vi "TekAFG3102.vi"() -> ()   [LabVIEW 2015]
uses:
  NetworkStream/NetworkStreamReceiverState.ctl
  Shared program Control/loop state machine.ctl
  NetworkStream/NetworkStreamStateMachineVariable.ctl
  NetworkStream/NetworkStreamData.ctl
  Shared program Control/MasterStatus.ctl
  <vilib>/dex/Stream Element Allocation Mode.ctl
  ICcamera/MyToolsFunction.lvlib
  Tek shared libraries/ArbitraryFunctions.lvlib
  NetworkStream/NetworkStream.lvlib
  Shared program Control/MySharedVariables.lvlib
panel:
  out "sequence number":u64
  out "loop state machine":T1=enum."load user waveform"
  in  "Stop Button":bool
  in  "slot to load (update first)":i32(ring) items=["Slot 1", "Slot 2", "Slot 3", "Slot 4"]
  in  "channels":enum32{"active channel", ""}(radio)
  in  "Channel ON/OFF":bool
  out "Network Stream State Indicator":T2
  out "Session Hash":u64
  out "ready":bool=TRUE
  in  "force trigger":bool
  in  "user waveform":bool
  in  "Tab Control":enum32{"CW", "AM", "FM", "PM", "Sweep", "Burst"}(tab)
  in  "CM cluster":T3={"Frequency (Hz)"=80000000.0, "Amplitude (V)"=0.2, "Phase (°)"=0.0, "Offset (Volt)"=0.0, "Standard waveform (1: Sine)"=1, "output mode"=0, "Modulation Waveform (1: Sine)"=1} {"Modulation Waveform (1: Sine)" items=["Sine"=1, "Square"=2, "Triangle"=3, "Ramp Up"=4, "Ramp Down"=5, "Noise"=100, "Arbitrary User1"=200, "Arbitrary User2"=201, "Arbitrary User3"=202, "Arbitrary User4"=203, "Edit Memory"=204]; "output mode" items=["Standard Function", "Arbitrary Waveform"]; "Standard waveform (1: Sine)" items=["Sine"=1, "Square"=2, "Pulse"=1002, "Ramp"=1001, "Noise"=1003, "DC"=6, "Sin(x)/x"=1004, "Gaussian"=1005, "Lorentz"=1006, "Exponential Rise"=1007, "Exponential Decay"=1008, "Haversine"=1009]}
  in  "AM Modulation Mode Cluster":T4={"waveform (1: Sine)"=1, "depth M (%)"=50.0, "Modulation source"=0, "AM Frequency (Hz)"=10.0, "ON/OFF"=FALSE} {"Modulation source" items=["Intern", "Extern"]; "waveform (1: Sine)" items=["Sine"=1, "Square"=2, "Pulse"=1002, "Ramp"=1001, "Noise"=1003, "DC"=6, "Sin(x)/x"=1004, "Gaussian"=1005, "Lorentz"=1006, "Exponential Rise"=1007, "Exponential Decay"=1008, "Haversine"=1009]}
  in  "FM":T5={"ON/OFF"=FALSE, "source (0: Internal)"=0, "peak deviation (1000000)"=1000000.0, "modulation frequency (10000)"=10000.0, "waveform (1: Sine)"=1} {"waveform (1: Sine)" items=["Sine"=1, "Square"=2, "Pulse"=1002, "Ramp"=1001, "Noise"=1003, "DC"=6, "Sin(x)/x"=1004, "Gaussian"=1005, "Lorentz"=1006, "Exponential Rise"=1007, "Exponential Decay"=1008, "Haversine"=1009]; "source (0: Internal)" items=["Internal", "External"]}
  in  "PM Modulation Cluster":T6={"Source (0: Internal)"=0, "Peak Deviation (90)"=90.0, "ON/OFF"=FALSE, "Modulation Frequency (10000)"=10000.0, "Modulation Waveform (1: Sine)"=1} {"Modulation Waveform (1: Sine)" items=["Sine"=1, "Square"=2, "Triangle"=3, "Ramp Up"=4, "Ramp Down"=5, "Noise"=100, "Arbitrary User1"=200, "Arbitrary User2"=201, "Arbitrary User3"=202, "Arbitrary User4"=203, "Edit Memory"=204]; "Source (0: Internal)" items=["Internal", "External"]}
  in  "resource name":refnum<k15>
  # "By default, Define User Waveform will assume \na modulation frequency = PM. However, the \nvalue has no effect on sent data to controlor and \nis purely arbitrary"
  # "Depth M is varied between 0% and 120% (the latter corresponding \nto a maximum amplitude of A(Vpp)). Cf p63 doc"
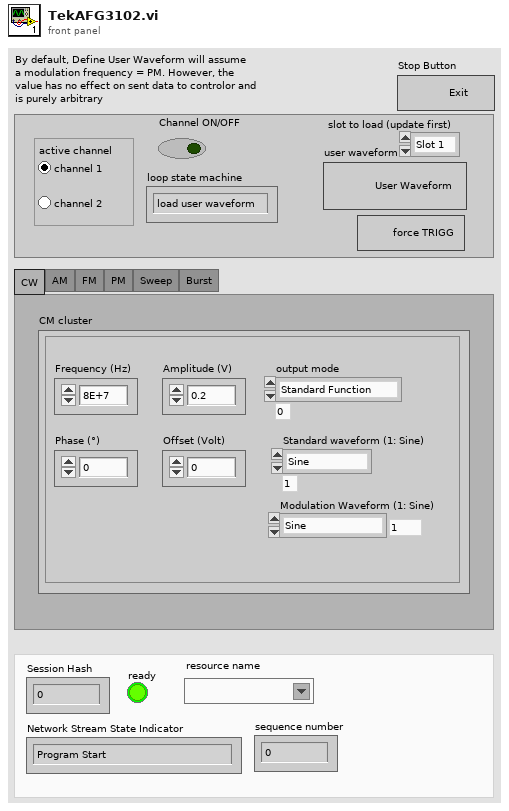
[diagram p1: front panel]
types:
  T1 = typedef "loop state machine.ctl" = enum16{"ready", "write on VISA", "get tek param", "load user waveform", "update channel parameters", "update status", "channel on/off", "initialize", "exit", "error"}
  T2 = typedef "NetworkStream.lvlib/NetworkStreamReceiverState.ctl" = enum16{"Program Start", "Waiting for connection", "Connected", "Connection lost", "Exit", "Unhandled Exception"}
  T3 = cluster{"Frequency (Hz)":dbl, "Amplitude (V)":dbl, "Phase (°)":dbl, "Offset (Volt)":dbl, "Standard waveform (1: Sine)":i32, "output mode":i32, "Modulation Waveform (1: Sine)":i32}
  T4 = cluster{"waveform (1: Sine)":i32, "depth M (%)":dbl, "Modulation source":u16, "AM Frequency (Hz)":dbl, "ON/OFF":bool}
  T5 = cluster{"ON/OFF":bool, "source (0: Internal)":i32, "peak deviation (1000000)":dbl, "modulation frequency (10000)":dbl, "waveform (1: Sine)":i32}
  T6 = cluster{"Source (0: Internal)":i32, "Peak Deviation (90)":dbl, "ON/OFF":bool, "Modulation Frequency (10000)":dbl, "Modulation Waveform (1: Sine)":i32}
  T7 = typedef "MySharedVariables.lvlib/MasterStatus.ctl" = cluster{"Camera done":bool, "Tektronik done":bool, "Motors done":bool, "Gage done":bool}[]
  T8 = typedef "NetworkStream.lvlib/NetworkStreamData.ctl" = cluster{"Command/Status":string, "Data":variant, "Session Hash":u64, "Sequence Number":u64}
  T9 = typedef "NetworkStream.lvlib/NetworkStreamStateMachineVariable.ctl" = cluster{"Network Stream Reader Endpoint":refnum<k21>, "Last Received Sequence Number":u64}
  T10 = cluster{"Frequency (Hz)":dbl, "Amplitude (V)":dbl, "Phase (°)":dbl, "Offset (Volt)":dbl, "waveform (1: Sine)":i32, "output mode":i32}
  T11 = cluster{"max number of waveforms":i32, "waveform quantum":i32, "max waveform size":i32, "min waveform size":i32}
  T12 = cluster{"Camera done":bool, "Tektronik done":bool, "Motors done":bool, "Gage done":bool}
  T13 = typedef "Stream Element Allocation Mode.ctl" = u32
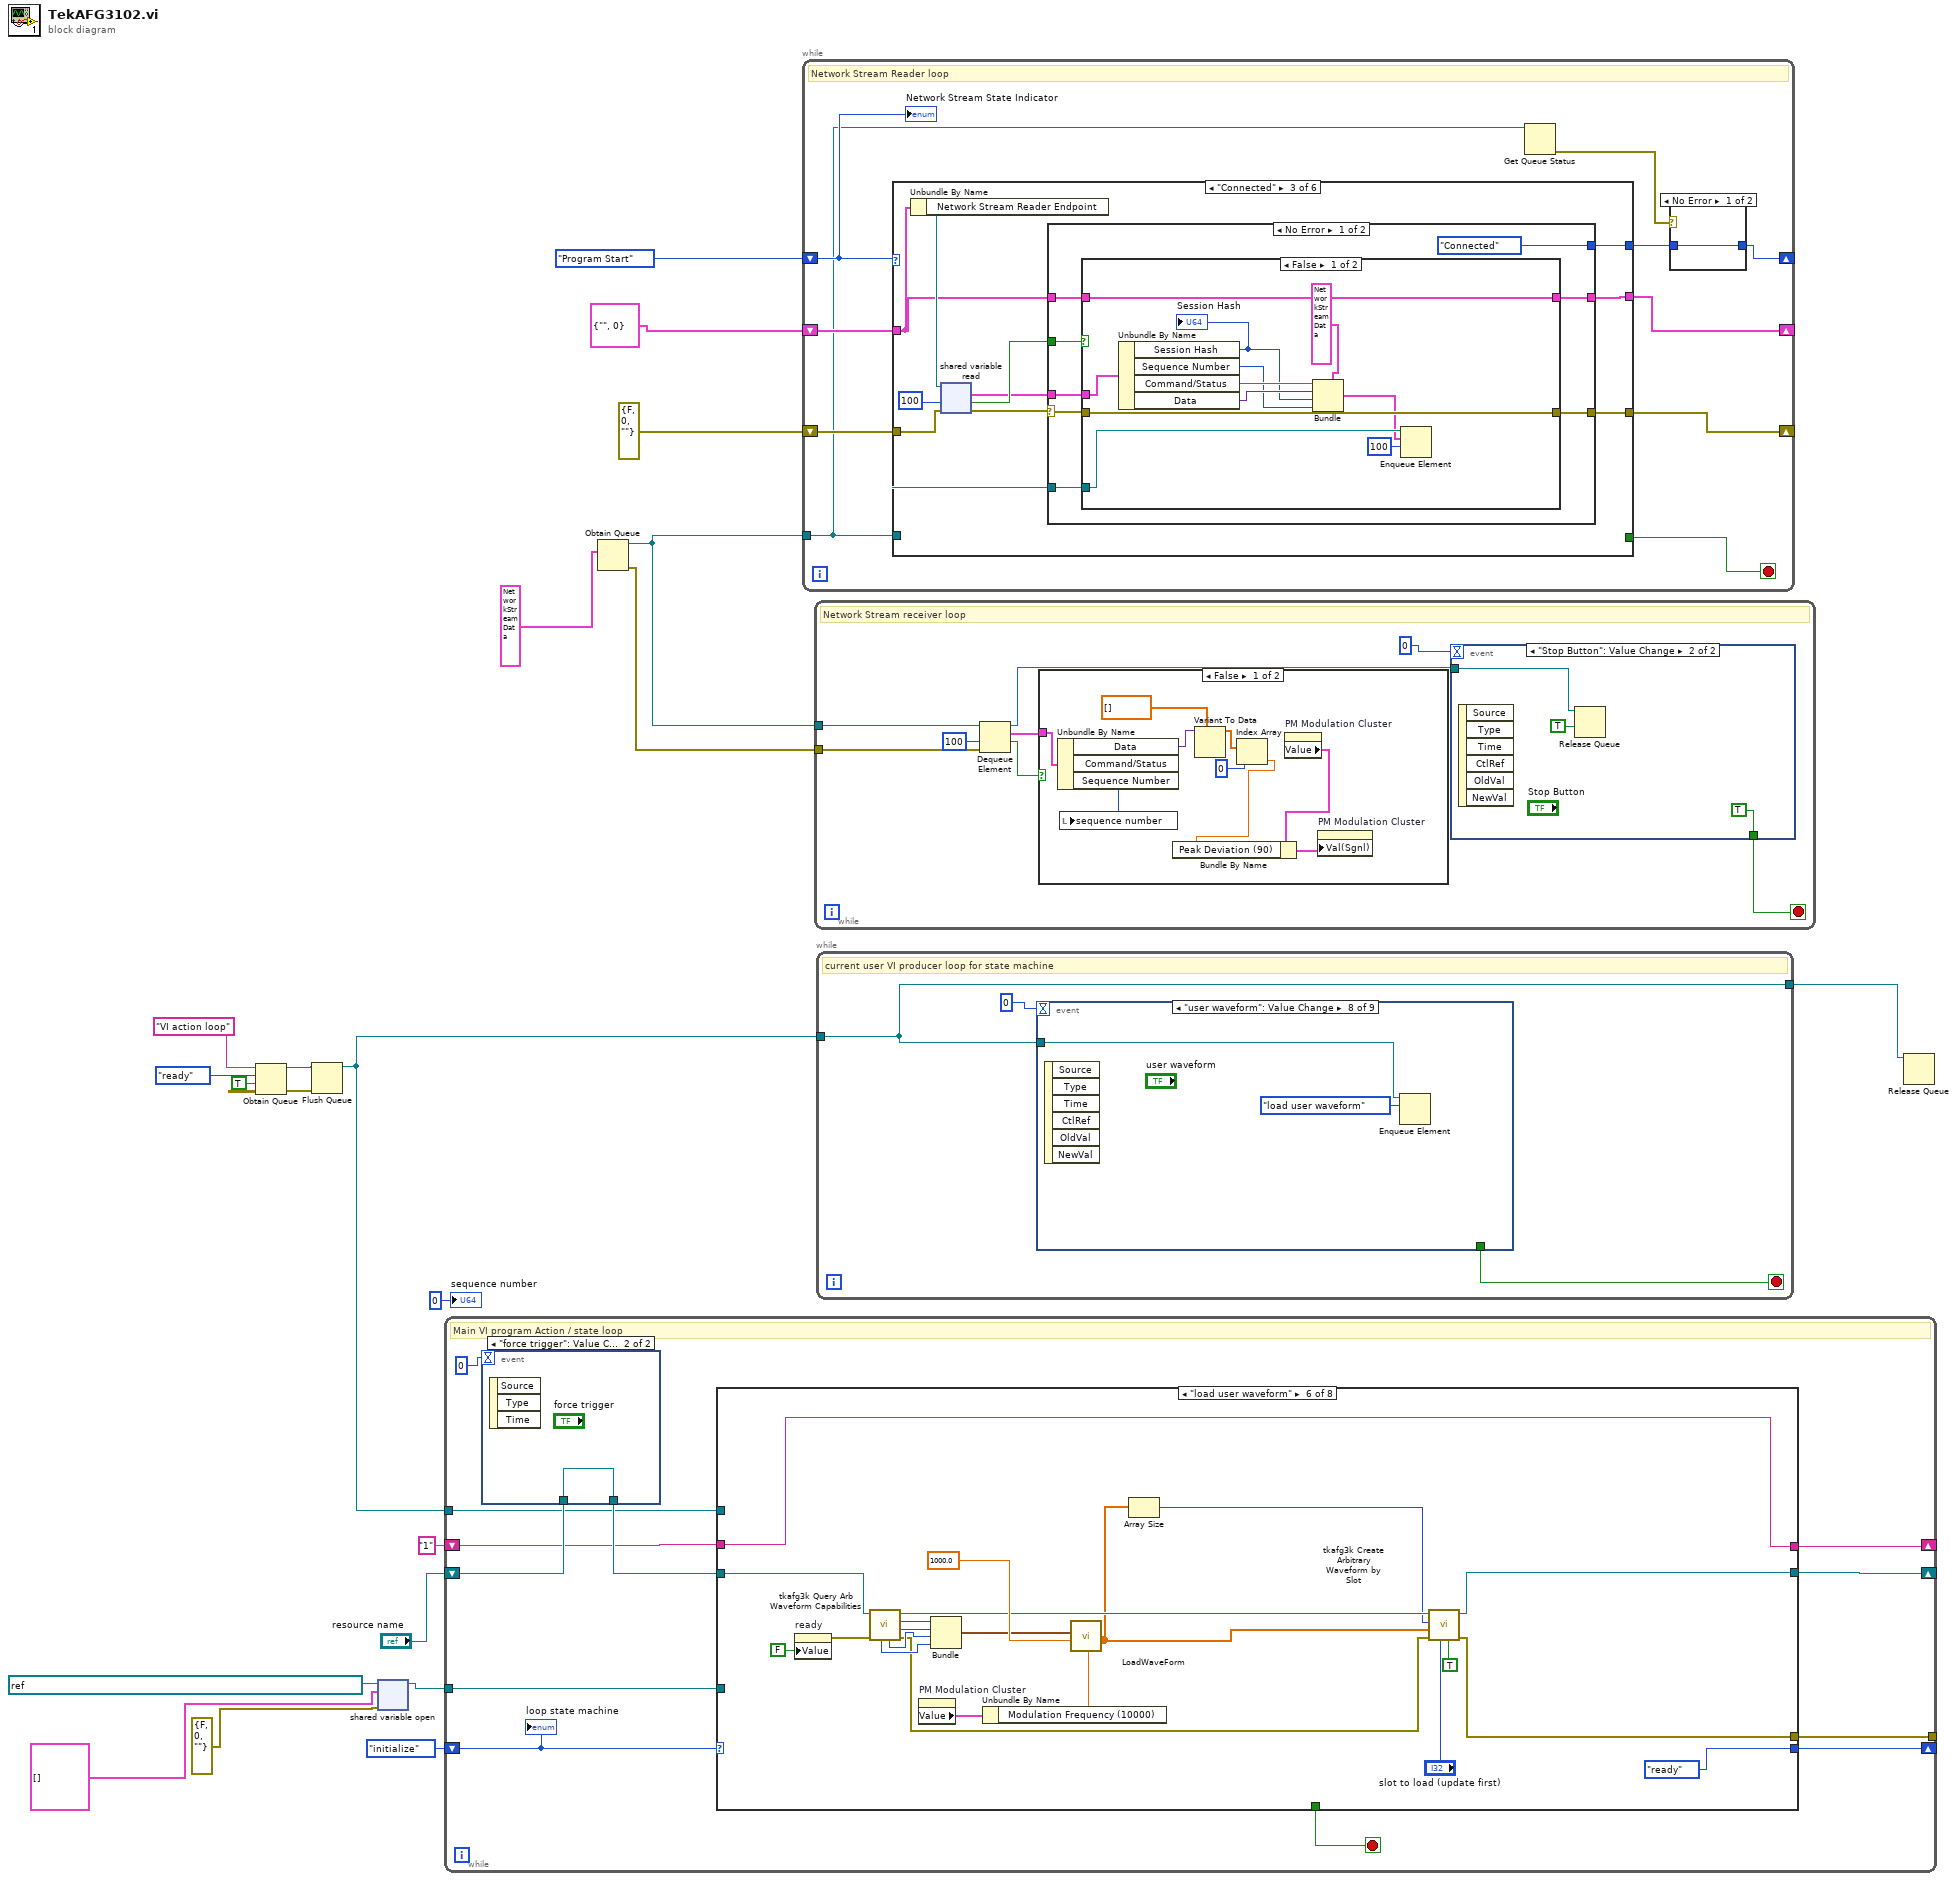
[diagram p0: block diagram]
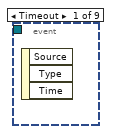
[diagram p2: hidden frame]
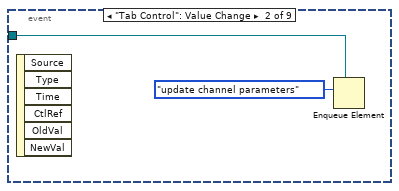
[diagram p3: hidden frame]
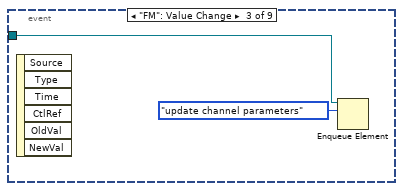
[diagram p4: hidden frame]
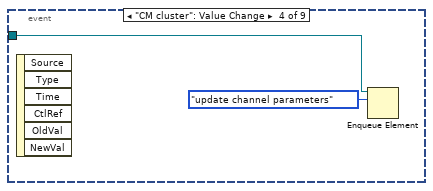
[diagram p5: hidden frame]
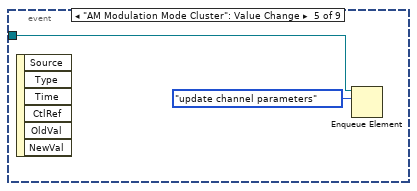
[diagram p6: hidden frame]
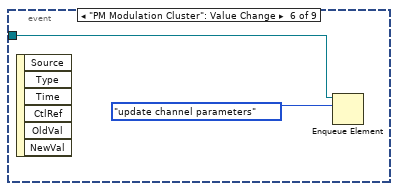
[diagram p7: hidden frame]
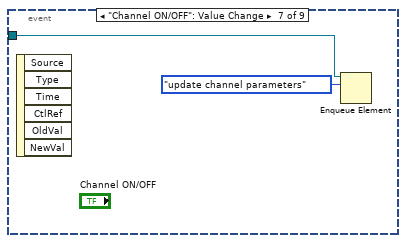
[diagram p8: hidden frame]
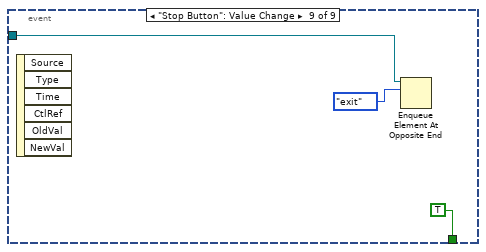
[diagram p9: hidden frame]
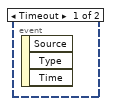
[diagram p11: hidden frame]
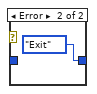
[diagram p12: hidden frame]
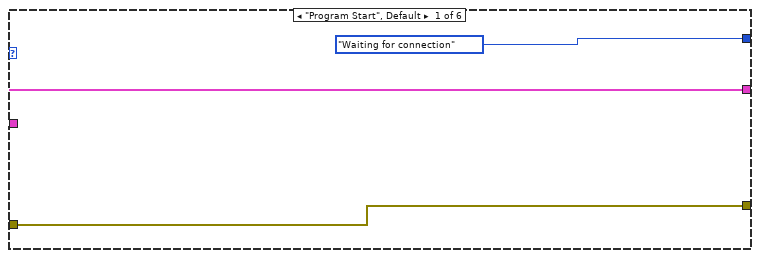
[diagram p13: hidden frame]
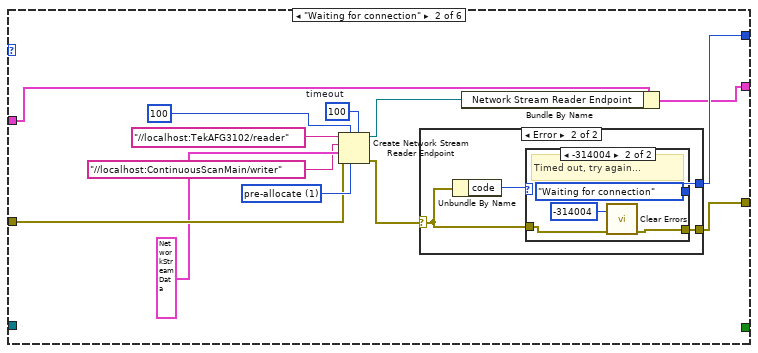
[diagram p14: hidden frame]
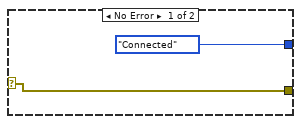
[diagram p15: hidden frame]
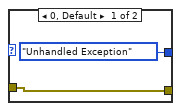
[diagram p16: hidden frame]
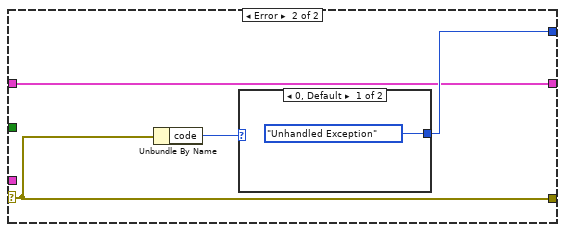
[diagram p18: hidden frame]
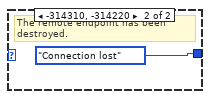
[diagram p19: hidden frame]
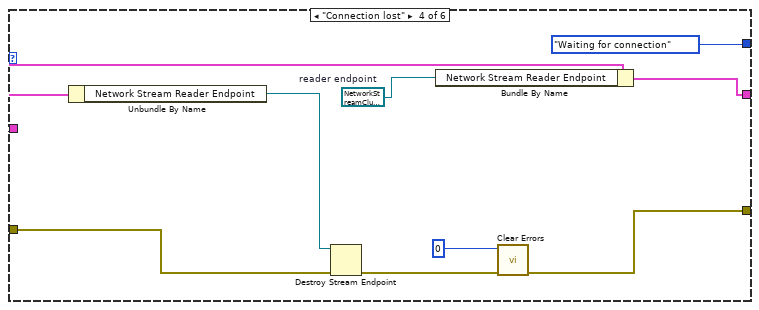
[diagram p20: hidden frame]
diagram:
  n1 = Obtain Queue(name (unnamed)="VI action loop", element data type=loop_state_machine."ready" ("loop state machine"), create if not found? (T)=TRUE) -> (queue out=w8:refnum<queue>, error out=w6:errorcluster)  [unwired: 2 in, 1 out]
  n2 = Flush Queue(queue=w8, error in (no error)=w6) -> (queue out=w7:refnum<queue>)  [unwired: 2 out]
  n3 = shared-variable-open(refnum<k21> "ni.var.psp://localhost/MySharedVariables/MasterStatusShared" ("shared variable refnum in"), errorcluster {"status"=FALSE, "code"=0, "source"=""} ("error in (no error)"), T7 [] ("MasterStatusShared")) -> (w3:refnum<k21>)  [unwired: 1 in, 1 out]
  n4 = while {
    tunnel: [w32] -> _
    shift-right: [w31] -> _
    shift-left: "resource name" -> [w26]
    shift-right: [w29] -> _
    shift-left: loop_state_machine."initialize" ("loop state machine") -> [w30]
    shift-right: [w27] -> _
    shift-left: "1" -> [w24]
    tunnel: w7 -> [w23]
    tunnel: w3 -> [w22]
    stop <- w33 stop-if-true
    # "Main VI program Action / state loop"
    n5 = event shown="[1] \"force trigger\": Value Change" {
      selector: _ -> [_ _]
      dyn-events: _ -> [_ _]
      timeout: 0 -> [_ _]
      tunnel: w26 -> [w34 w36]
      tunnel: [w34 w36] -> w25
      event Timeout {
        n6 = event-data() -> ()  [unwired: 1 in, 3 out]
        "ready" <- TRUE
      }
      event "force trigger": Value Change {
        n7 = event-data() -> ()  [unwired: 1 in, 3 out]
      }
    }
    n8 = case shown="\"load user waveform\"" w30 {
      tunnel: [_ TRUE _ _ _ _ _ _] -> w33
      tunnel: [w41 w54 errorcluster {"status"=FALSE, "code"=0, "source"=""} ("error out") errorcluster {"status"=FALSE, "code"=0, "source"=""} ("error out") w74 w134 w150 errorcluster {"status"=FALSE, "code"=0, "source"=""} ("error out")] -> w32
      tunnel: [w38 w55 w66 w71 w77 w133 w153 w159] -> w31
      tunnel: [w42 loop_state_machine."exit" ("loop state machine") w63 loop_state_machine."exit" ("loop state machine") loop_state_machine."update status" ("loop state machine") loop_state_machine."ready" ("loop state machine") loop_state_machine."ready" ("loop state machine") loop_state_machine."ready" ("loop state machine")] -> w29
      tunnel: w25 -> [w40 w55 w66 w71 w78 w144 w154 w159]
      tunnel: [w37 w52 w65 w72 w76 w132 w152 w160] -> w27
      tunnel: w24 -> [w37 w52 w65 w72 _ w132 w152 w160]
      tunnel: w23 -> [_ _ w59 _ _ _ _ _]
      tunnel: w22 -> [_ w51 _ _ _ _ _ w156]
      frame "initialize", Default {
        n9 = call <instrlib>:"tkafg3k Initialize.vi"("error in (no error)"=errorcluster {"status"=FALSE, "code"=0, "source"=""}, "resource name"=w40) -> ("error out"=w45:errorcluster, "instrument handle out"=w43:refnum<k15>)  [unwired: 8 in]
        n10 = call <instrlib>:"tkafg3k Clear Arbitrary Waveform.vi"("error in (no error)"=w45, "waveform handle"=-1, "instrument handle"=w43) -> ("error out"=w41:errorcluster, "instrument handle out"=w39:refnum<k15>)  [unwired: 7 in]
        n11 = case shown="Error" w41 {
          tunnel: [loop_state_machine."update channel parameters" ("loop state machine") loop_state_machine."exit" ("loop state machine")] -> w42
          tunnel: w39 -> [w47 w49]
          tunnel: [w47 w49] -> w38
          frame No Error {
          }
          frame Error {
          }
        }
      }
      frame "exit" {
        n12 = Close Variable Connection(11:w51) -> ()  [unwired: 1 in, 1 out]
        n13 = call <instrlib>:"tkafg3k Close.vi"("instrument handle"=w55) -> ("error out"=w56:errorcluster)  [unwired: 10 in]
        n14 = call <vilib>:"Simple Error Handler.vi"("error in (no error)"=w56) -> ("error out"=w54:errorcluster)  [unwired: 1 in, 7 out]
      }
      frame "ready" {
        n15 = Get Queue Status(queue=w59) -> (queue out=w58:refnum<queue>)  [unwired: 2 in, 7 out]
        n16 = Dequeue Element(queue=w58, timeout in ms (-1)=200) -> (element=w61:T1, error out=w62:errorcluster)  [unwired: 1 in, 2 out]
        n17 = case shown="No Error" w62 {
          tunnel: [w67 loop_state_machine."exit" ("loop state machine")] -> w63
          tunnel: w61 -> [w67 _]
          frame No Error {
          }
          frame Error {
          }
        }
      }
      frame "error" {
      }
      frame "update channel parameters" {
        n18 = case shown="\"active channel\", Default" "channels" {
          tunnel: ["1" "2"] -> w79
          frame "active channel", Default {
            n19 = property on="ready" class="Bool (strict)"("Value"=FALSE ("ready")) -> ()  [unwired: 2 in, 2 out]
          }
          frame "" {
            n20 = property on="ready" class="Bool (strict)"("Value"=FALSE ("ready")) -> ()  [unwired: 2 in, 2 out]
          }
        }
        n21 = case shown="\"PM\"" "Tab Control" {
          tunnel: w79 -> [w81 w90 w98 w106 w111 w116]
          tunnel: w78 -> [w88 w97 w105 w110 w115 w122]
          tunnel: [w84 w92 w100 w109 w113 w118] -> w77
          tunnel: [w86 w94 w102 w108 w112 w120] -> w74
          tunnel: [w81 w90 w98 w106 w111 w116] -> w76
          frame "CW", Default {
            w89 = 0 items=["Continuous"=0, "Modulation"=1001, "Sweep"=1002, "Burst"=1] ("operation mode (0: Continuous)")
            n22 = call <instrlib>:"tkafg3k Configure Operation Mode.vi"("operation mode (0: Continuous)"=w89, "channel name (\"1\")"=w81, "instrument handle"=w88) -> ("error out"=w87:errorcluster, "instrument handle out"=w85:refnum<k15>)  [unwired: 7 in]
            n23 = call "Update_CW.vi"("channel name (\"1\")"=w81, "error in (no error)"=w87, "CM cluster"="CM cluster", "resource name"=w85) -> ("error out"=w86:errorcluster, "output cluster"=w82:T10, "instrument handle out"=w84:refnum<k15>)  [unwired: 5 in]
            n24 = Unbundle By Name(w82) -> ()  [unwired: 1 out]
          }
          frame "FM" {
            w96 = 1001 items=["Continuous"=0, "Modulation"=1001, "Sweep"=1002, "Burst"=1] ("operation mode (0: Continuous)")
            n25 = call <instrlib>:"tkafg3k Configure Operation Mode.vi"("operation mode (0: Continuous)"=w96, "channel name (\"1\")"=w90, "instrument handle"=w97) -> ("error out"=w95:errorcluster, "instrument handle out"=w93:refnum<k15>)  [unwired: 7 in]
            n26 = call "Update_FM.vi"("error in (no error)"=w95, "channel name (\"1\")"=w90, "FM"="FM", "resource name"=w93) -> ("error out"=w94:errorcluster, "instrument handle out"=w92:refnum<k15>)  [unwired: 5 in, 1 out]
          }
          frame "PM" {
            w104 = 1001 items=["Continuous"=0, "Modulation"=1001, "Sweep"=1002, "Burst"=1] ("operation mode (0: Continuous)")
            n27 = call <instrlib>:"tkafg3k Configure Operation Mode.vi"("operation mode (0: Continuous)"=w104, "channel name (\"1\")"=w98, "instrument handle"=w105) -> ("error out"=w103:errorcluster, "instrument handle out"=w101:refnum<k15>)  [unwired: 7 in]
            n28 = call "Update_PM.vi"("PM Modulation Cluster"="PM Modulation Cluster", "error in (no error)"=w103, "channel name (\"1\")"=w98, "resource name"=w101) -> ("error out"=w102:errorcluster, "instrument handle out"=w100:refnum<k15>)  [unwired: 5 in, 1 out]
          }
          frame "Sweep" {
            w107 = 1002 items=["Continuous"=0, "Modulation"=1001, "Sweep"=1002, "Burst"=1] ("operation mode (0: Continuous)")
            n29 = call <instrlib>:"tkafg3k Configure Operation Mode.vi"("operation mode (0: Continuous)"=w107, "channel name (\"1\")"=w106, "instrument handle"=w110) -> ("error out"=w108:errorcluster, "instrument handle out"=w109:refnum<k15>)  [unwired: 7 in]
          }
          frame "Burst" {
            w114 = 1 items=["Continuous"=0, "Modulation"=1001, "Sweep"=1002, "Burst"=1] ("operation mode (0: Continuous)")
            n30 = call <instrlib>:"tkafg3k Configure Operation Mode.vi"("operation mode (0: Continuous)"=w114, "channel name (\"1\")"=w111, "instrument handle"=w115) -> ("error out"=w112:errorcluster, "instrument handle out"=w113:refnum<k15>)  [unwired: 7 in]
          }
          frame "AM" {
            w123 = 1001 items=["Continuous"=0, "Modulation"=1001, "Sweep"=1002, "Burst"=1] ("operation mode (0: Continuous)")
            n31 = call <instrlib>:"tkafg3k Configure Operation Mode.vi"("operation mode (0: Continuous)"=w123, "channel name (\"1\")"=w116, "instrument handle"=w122) -> ("error out"=w121:errorcluster, "instrument handle out"=w119:refnum<k15>)  [unwired: 7 in]
            n32 = call "Update_AM.vi"("AM Modulation Mode Cluster"="AM Modulation Mode Cluster", "error in (no error)"=w121, "channel name (\"1\")"=w116, "resource name"=w119) -> ("error out"=w120:errorcluster, "instrument handle out"=w118:refnum<k15>)  [unwired: 5 in, 1 out]
          }
        }
      }
      frame "load user waveform" {
        n33 = property on="ready" class="Bool (strict)"("Value"=FALSE ("ready")) -> (error out=w130:errorcluster)  [unwired: 2 in, 1 out]
        n34 = call <instrlib>:"tkafg3k Query Arb Waveform Capabilities.vi"("error in (no error)"=w130, "instrument handle"=w144) -> ("error out"=w137:errorcluster, "waveform quantum"=w148:i32, "max number of waveforms"=w147:i32, "instrument handle out"=w138:refnum<k15>, "max waveform size"=w143:i32, "min waveform size"=w142:i32)  [unwired: 4 in]
        n35 = property on="PM Modulation Cluster" class="Clust (strict)"() -> ("Value"=w129:T6)  [unwired: 2 in, 2 out]
        n36 = Bundle("max number of waveforms"=w147, "waveform quantum"=w148, "max waveform size"=w143, "min waveform size"=w142) -> (w141:T11)  [unwired: 1 in]
        n37 = Unbundle By Name(w129) -> ("Modulation Frequency (10000)"=w128:dbl)
        n38 = call "LoadWaveForm.vi"("modulation frequency (Hz)"=w128, "Npoint"=1000.0 ("arbitrary frequency (Npoints)"), "arbitrary parameters"=w141) -> ("waveform"=w131:dbl[])  [unwired: 8 in]
        n39 = Array Size(array=w131) -> (size(s)=w136:i32)
        n40 = call <instrlib>:"tkafg3k Create Arbitrary Waveform by Slot.vi"("overwrite (False)"=TRUE, "slot (0: Slot 1)"="slot to load (update first)", "error in (no error)"=w137, "waveform data array"=w131, "waveform size (1000)"=w136, "instrument handle"=w138) -> ("error out"=w134:errorcluster, "instrument handle out"=w133:refnum<k15>)  [unwired: 4 out]
      }
      frame "channel on/off" {
        n41 = property on="Channel ON/OFF" class="Bool (strict)"() -> ("Value"=w151:bool)  [unwired: 2 in, 2 out]
        n42 = call <instrlib>:"tkafg3k Configure Output Enabled.vi"("channel enabled (True)"=w151, "channel name (\"1\")"=w152, "instrument handle"=w154) -> ("error out"=w150:errorcluster, "instrument handle out"=w153:refnum<k15>)  [unwired: 7 in]
      }
      frame "update status" {
        n43 = property on="Network Stream State Indicator" class="Enum (strict)"() -> ("Value"=w155:T2)  [unwired: 2 in, 2 out]
        n44 = case shown="\"Connected\"" w155 {
          tunnel: w156 -> [_ w166]
          frame "Program Start", Default {
          }
          frame "Connected" {
            n45 = local read "sequence number"() -> (w164:u64)
            n46 = shared-variable-read(w166) -> (w168:refnum<k21>, w165:T7)  [unwired: 1 in, 2 out]
            n47 = Index Array(array=w165, index=w164) -> (element=w163:T12)
            n48 = Bundle By Name(cluster=w163, "Tektronik done"=TRUE) -> (w162:T12)
            n49 = Replace Array Subset(array=w165, new element=w162, index=w164) -> (w167:T7)
            n50 = shared-variable-write(w168, w167) -> ()  [unwired: 1 in, 2 out]
          }
        }
      }
    }
    "loop state machine" <- w30
  }
  n51 = Obtain Queue(element data type=T8 {"Command/Status"="", "Data"=variant, "Session Hash"=0, "Sequence Number"=0} ("NetworkStreamCluster")) -> (queue out=w17:refnum<queue>, error out=w18:errorcluster)  [unwired: 4 in, 1 out]
  n52 = while {
    shift-right: [w176] -> _
    shift-left: T9 {"Network Stream Reader Endpoint"="", "Last Received Sequence Number"=0} ("StateMachineVariable") -> [w178]
    shift-right: [w171] -> _
    shift-left: NetworkStreamReceiverState."Program Start" -> [w177]
    shift-right: [w175] -> _
    shift-left: errorcluster {"status"=FALSE, "code"=0, "source"=""} ("error in (no error)") -> [w173]
    tunnel: w17 -> [w169]
    stop <- w174 stop-if-true
    # "Network Stream Reader loop"
    n53 = case shown="\"Connected\"" w177 {
      tunnel: [NetworkStreamReceiverState."Waiting for connection" w192 w214 NetworkStreamReceiverState."Waiting for connection" NetworkStreamReceiverState."Exit" NetworkStreamReceiverState."Exit"] -> w172
      tunnel: [w182 w191 w215 w251 w264 w272] -> w175
      tunnel: [w181 w190 w212 w247 w257 w269] -> w176
      tunnel: [_ _ _ _ TRUE _] -> w174
      tunnel: w178 -> [w181 w188 w211 w248 w258 w269]
      tunnel: w173 -> [w182 w187 w210 w250 w259 w270]
      tunnel: w169 -> [_ _ w209 _ _ _]
      frame "Program Start", Default {
      }
      frame "Waiting for connection" {
        w189 = T13 1 items=["allocate as needed", "pre-allocate"] ("element allocation mode")
        w196 = 100  # timeout
        n54 = Create Network Stream Reader Endpoint(5:w196, 6:w189, 7:100 ("reader buffer size"), 8:w187, 9:T8 {"Command/Status"="", "Data"=variant, "Session Hash"=0, "Sequence Number"=0} ("NetworkStreamCluster"), 10:"//localhost:ContinuousScanMain/writer" ("writer url"), 11:"//localhost:TekAFG3102/reader" ("reader name")) -> (0:w193:errorcluster, 3:w185:refnum<k21>)
        n55 = case shown="Error" w193 {
          selector: w193 -> [w197 w200]
          tunnel: [NetworkStreamReceiverState."Connected" w202] -> w192
          tunnel: [w197 w199] -> w191
          frame No Error {
          }
          frame Error {
            n56 = Unbundle By Name(w200) -> ("code"=w201:i32)
            n57 = case shown="-314004" w201 {
              tunnel: [NetworkStreamReceiverState."Unhandled Exception" NetworkStreamReceiverState."Waiting for connection"] -> w202
              tunnel: w200 -> [w203 w206]
              tunnel: [w203 w205] -> w199
              frame 0, Default {
              }
              frame -314004 {
                # "Timed out, try again..."
                n58 = call <vilib>:"Clear Errors.vi"("error in (no error)"=w206, "specific error code to clear (0: all)"=-314004) -> ("error out"=w205:errorcluster)  [unwired: 4 in, 1 out]
              }
            }
          }
        }
        n59 = Bundle By Name(cluster=w188, "Network Stream Reader Endpoint"=w185) -> (w190:T9)
      }
      frame "Connected" {
        n60 = Unbundle By Name(w211) -> ("Network Stream Reader Endpoint"=w213:refnum<k21>)
        n61 = shared-variable-read(w213, w210, 100 ("timeout ms (-1)")) -> (w216:errorcluster, w218:bool, w217:T8)  [unwired: 1 out]
        n62 = case shown="No Error" w216 {
          selector: w216 -> [w225 w244]
          tunnel: w218 -> [w227 _]
          tunnel: w217 -> [w226 _]
          tunnel: [w224 w244] -> w215
          tunnel: [NetworkStreamReceiverState."Connected" w242] -> w214
          tunnel: [w222 w241] -> w212
          tunnel: w211 -> [w221 w241]
          tunnel: w209 -> [w220 _]
          frame No Error {
            n63 = case shown="False" w227 {
              tunnel: [w234 w240] -> w224
              tunnel: w225 -> [w234 w240]
              tunnel: w226 -> [w238 _]
              tunnel: [w235 w239] -> w222
              tunnel: w221 -> [w235 w239]
              tunnel: w220 -> [w233 _]
              frame False {
                n64 = Unbundle By Name(w238) -> ("Session Hash"=w230:u64, "Sequence Number"=w229:u64, "Command/Status"=w237:string, "Data"=w236:variant)
                "Session Hash" <- w230
                n65 = Bundle(cluster=T8 {"Command/Status"="", "Data"=variant, "Session Hash"=0, "Sequence Number"=0} ("NetworkStreamCluster"), "Command/Status"=w237, "Data"=w236, "Session Hash"=w230, "Sequence Number"=w229) -> (w232:T8)
                n66 = Enqueue Element(queue=w233, element=w232, timeout in ms (-1)=100) -> ()  [unwired: 1 in, 3 out]
              }
              frame True {
              }
            }
          }
          frame Error {
            n67 = Unbundle By Name(w244) -> ("code"=w243:i32)
            n68 = case shown="0, Default" w243 {
              tunnel: [NetworkStreamReceiverState."Unhandled Exception" NetworkStreamReceiverState."Connection lost"] -> w242
              frame 0, Default {
              }
              frame -314310, -314220 {
                # "The remote endpoint has been destroyed."
              }
            }
          }
        }
      }
      frame "Connection lost" {
        w254 = refnum<k21> refnum  # reader endpoint
        n69 = Unbundle By Name(w248) -> ("Network Stream Reader Endpoint"=w249:refnum<k21>)
        n70 = Destroy Stream Endpoint(8:w250, 11:w249) -> (0:w253:errorcluster)
        n71 = Bundle By Name(cluster=w248, "Network Stream Reader Endpoint"=w254) -> (w247:T9)
        n72 = call <vilib>:"Clear Errors.vi"("error in (no error)"=w253, "specific error code to clear (0: all)"=0) -> ("error out"=w251:errorcluster)  [unwired: 4 in, 1 out]
      }
      frame "Exit" {
        w260 = refnum<k21> refnum  # reader endpoint
        n73 = Unbundle By Name(w258) -> ("Network Stream Reader Endpoint"=w256:refnum<k21>)
        n74 = Not Equal?(x=w260, y=w256) -> (x != y?=w262:bool)
        n75 = case shown="True" w262 {
          tunnel: [w265 w268] -> w264
          tunnel: w259 -> [w265 w267]
          tunnel: w256 -> [_ w266]
          frame False {
          }
          frame True {
            n76 = Destroy Stream Endpoint(8:w267, 11:w266) -> (0:w268:errorcluster)
          }
        }
        n77 = Bundle By Name(cluster=w258, "Network Stream Reader Endpoint"=w260) -> (w257:T9)
      }
      frame "Unhandled Exception" {
        n78 = call <vilib>:"General Error Handler.vi"("error in (no error)"=w270) -> ("error out"=w272:errorcluster)  [unwired: 10 in, 4 out]
      }
    }
    n79 = Get Queue Status(queue=w169) -> (error out=w170:errorcluster)  [unwired: 2 in, 7 out]
    n80 = case shown="No Error" w170 {
      tunnel: w172 -> [w179 _]
      tunnel: [w179 NetworkStreamReceiverState."Exit"] -> w171
      frame No Error {
      }
      frame Error {
      }
    }
    "Network Stream State Indicator" <- w177
  }
  n81 = while {
    tunnel: w18 -> [w274]
    tunnel: w17 -> [w275]
    stop <- w280 stop-if-true
    # "Network Stream receiver loop"
    n82 = Dequeue Element(queue=w275, timeout in ms (-1)=100, error in (no error)=w274) -> (queue out=w276:refnum<queue>, element=w278:T8, timed out?=w273:bool)  [unwired: 1 out]
    n83 = case shown="False" w273 {
      tunnel: w278 -> [w289 _]
      frame False {
        n84 = Unbundle By Name(w289) -> ("Data"=w286:variant, "Sequence Number"=w288:u64)  [unwired: 1 out]
        n85 = local write "sequence number"(w288) -> ()
        n86 = Variant To Data(type=dbl[] [] ("subarray 2"), Variant=w286) -> (data=w285:dbl[])  [unwired: 1 in, 1 out]
        n87 = Index Array(array=w285, index=0) -> (element=w283:dbl)
        n88 = property on="PM Modulation Cluster" class="Clust (strict)"() -> ("Value"=w282:T6)  [unwired: 2 in, 2 out]
        n89 = Bundle By Name(cluster=w282, "Peak Deviation (90)"=w283) -> (w281:T6)
        n90 = property on="PM Modulation Cluster" class="Clust (strict)"("Val(Sgnl)"=w281) -> ()  [unwired: 2 in, 2 out]
      }
      frame True {
      }
    }
    n91 = event shown="[1] \"Stop Button\": Value Change" {
      selector: _ -> [_ _]
      dyn-events: _ -> [_ _]
      timeout: 0 -> [_ _]
      tunnel: [_ TRUE] -> w280
      tunnel: w276 -> [_ w291]
      event Timeout {
        n92 = event-data() -> ()  [unwired: 1 in, 3 out]
      }
      event "Stop Button": Value Change {
        n93 = event-data() -> ()  [unwired: 1 in, 6 out]
        n94 = Release Queue(queue=w291, force destroy? (F)=TRUE) -> ()  [unwired: 1 in, 3 out]
      }
    }
  }
  n95 = while {
    tunnel: w7 -> [w294]
    tunnel: [w294] -> w10
    stop <- w293 stop-if-true
    # "current user VI producer loop for state machine"
    n96 = event shown="[7] \"user waveform\": Value Change" {
      selector: _ -> [_ _ _ _ _ _ _ _ _]
      dyn-events: _ -> [_ _ _ _ _ _ _ _ _]
      timeout: 0 -> [_ _ _ _ _ _ _ _ _]
      tunnel: w294 -> [_ w297 w298 w300 w302 w304 w306 w308 w312]
      tunnel: [_ _ _ _ _ _ _ _ TRUE] -> w293
      event Timeout {
        n97 = event-data() -> ()  [unwired: 1 in, 3 out]
      }
      event "Tab Control": Value Change {
        n98 = event-data() -> ()  [unwired: 1 in, 6 out]
        n99 = Enqueue Element(queue=w297, element=loop_state_machine."update channel parameters") -> ()  [unwired: 2 in, 3 out]
      }
      event "FM": Value Change {
        n100 = event-data() -> ()  [unwired: 1 in, 6 out]
        n101 = Enqueue Element(queue=w298, element=loop_state_machine."update channel parameters") -> ()  [unwired: 2 in, 3 out]
      }
      event "CM cluster": Value Change {
        n102 = event-data() -> ()  [unwired: 1 in, 6 out]
        n103 = Enqueue Element(queue=w300, element=loop_state_machine."update channel parameters") -> ()  [unwired: 2 in, 3 out]
      }
      event "AM Modulation Mode Cluster": Value Change {
        n104 = event-data() -> ()  [unwired: 1 in, 6 out]
        n105 = Enqueue Element(queue=w302, element=loop_state_machine."update channel parameters") -> ()  [unwired: 2 in, 3 out]
      }
      event "PM Modulation Cluster": Value Change {
        n106 = event-data() -> ()  [unwired: 1 in, 6 out]
        n107 = Enqueue Element(queue=w304, element=loop_state_machine."update channel parameters") -> ()  [unwired: 2 in, 3 out]
      }
      event "Channel ON/OFF": Value Change {
        n108 = event-data() -> ()  [unwired: 1 in, 6 out]
        n109 = Enqueue Element(queue=w306, element=loop_state_machine."update channel parameters") -> ()  [unwired: 2 in, 3 out]
      }
      event "user waveform": Value Change {
        n110 = event-data() -> ()  [unwired: 1 in, 6 out]
        n111 = Enqueue Element(queue=w308, element=loop_state_machine."load user waveform") -> ()  [unwired: 2 in, 3 out]
      }
      event "Stop Button": Value Change {
        n112 = event-data() -> ()  [unwired: 1 in, 6 out]
        n113 = Enqueue Element At Opposite End(queue=w312, element=loop_state_machine."exit") -> ()  [unwired: 2 in, 3 out]
      }
    }
  }
  n114 = Release Queue(queue=w10) -> ()  [unwired: 2 in, 3 out]
  "sequence number" <- u64 0 ("sequence number")
